vi "Remove Vx.vi"(11 "Path in":path) -> (3 "Path out":path)   [LabVIEW 2015]
uses:
  <vilib>/regexp/Match Regular Expression.xnode
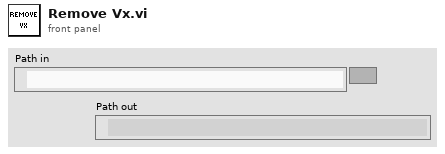
[diagram p1: front panel]
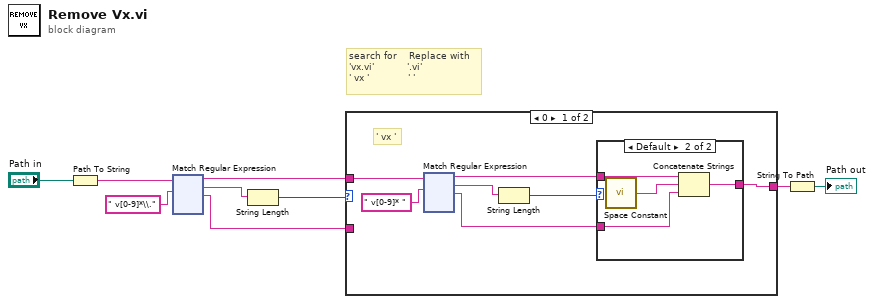
[diagram p0: block diagram]
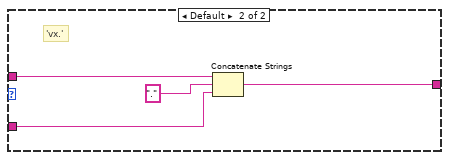
[diagram p3: hidden frame]
diagram:
  # "search for    Replace with\n'vx.vi'           '.vi'\n' vx '             ' '"
  n1 = Path To String(path="Path in") -> (string=w2:string)
  n2 = xnode "Match Regular Expression"("input string"=w2, "regular expression"=" v[0-9]*\\.") -> ("before match"=w6:string, "whole match"=w4:string, "after match"=w5:string)  [unwired: 4 in, 2 out]
  n3 = String Length(string=w4) -> (length=w3:i32)
  n4 = case shown="0" w3 {
    tunnel: w6 -> [w11 w138]
    tunnel: [w10 w137] -> w1
    tunnel: w5 -> [_ w136]
    frame 0 {
      # "' vx '"
      n5 = xnode "Match Regular Expression"("input string"=w11, "regular expression"=" v[0-9]* ") -> ("before match"=w15:string, "whole match"=w13:string, "after match"=w14:string)  [unwired: 4 in, 2 out]
      n6 = String Length(string=w13) -> (length=w12:i32)
      n7 = case shown="Default" w12 {
        tunnel: w15 -> [w17 w20]
        tunnel: [w17 w19] -> w10
        tunnel: w14 -> [_ w18]
        frame 0 {
        }
        frame Default {
          n8 = call <vilib>:"Space Constant.vi"() -> ("String"=w21:string)
          n9 = Concatenate Strings(w20, w21, w18) -> (w19:string)
        }
      }
    }
    frame Default {
      # "'vx.'"
      n10 = Concatenate Strings(w138, ".", w136) -> (w137:string)
    }
  }
  n11 = String To Path(string=w1) -> (path=→"Path out":path)
